vi "Show Module Diagram--helper.vi"(8 "error in (no error)":errorcluster, 11 "Module DQMH Path":path) -> (0 "error out":errorcluster)   [LabVIEW 2020, in "UI Manager.lvlib"]
doc: "____\nHAMPEL SOFTWARE ENGINEERING v2.6.0 (2023-12-19 10:54)"
uses:
  UI Manager.lvlib
  Libraries/hse-libraries/Source/hse-dqmh/hse-dqmh-dynamicrequesters.lvlib
  Libraries/hse-libraries/Source/hse-dqmh/hse-dqmh.lvlib
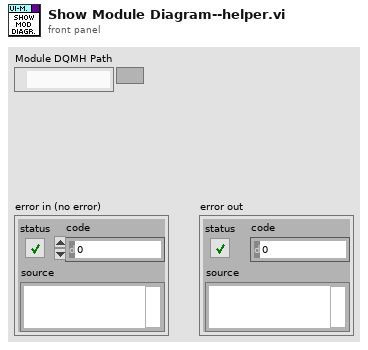
[diagram p1: front panel]
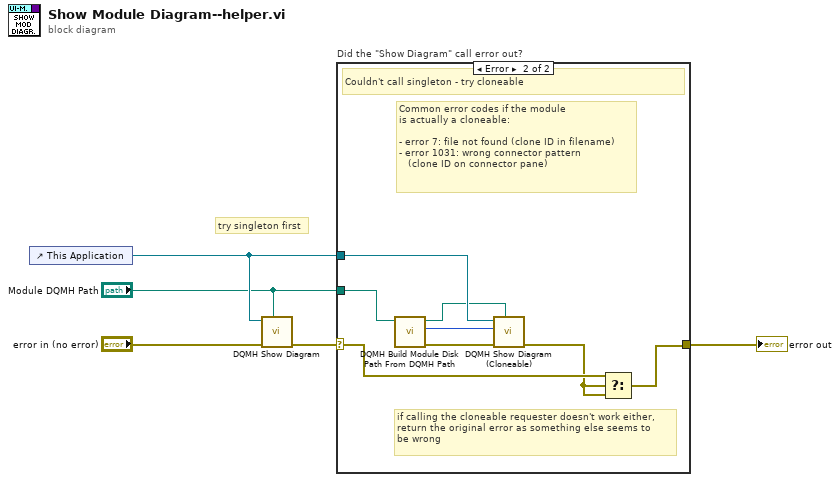
[diagram p0: block diagram]
diagram:
  # "try singleton first"
  n1 = control-ref of="This Application"() -> (w2:refnum<vi>)
  n2 = call "DQMH Show Diagram.vi"("Module Disk Path"="Module DQMH Path", "error in (no error)"="error in (no error)", "Application reference"=w2) -> ("error out"=w5:errorcluster)  [unwired: 8 in]
  n3 = case "Did the \"Show Diagram\" call error out?" shown="Error" w5 {
    selector: w5 -> [w6 w9]
    tunnel: "Module DQMH Path" -> [_ w13]
    tunnel: w2 -> [_ w14]
    tunnel: [w6 w8] -> w3
    frame No Error {
    }
    frame Error {
      # "if calling the cloneable requester doesn't work either,\nreturn the original error as something else seems to \nbe wrong"
      # "Common error codes if the module \nis actually a cloneable:\n\n- error 7: file not found (clone ID in filename)\n- error 1031: wrong connector pattern \n   (clone ID on connector pane)"
      # "Couldn't call singleton - try cloneable"
      n4 = call "DQMH Build Module Disk Path From DQMH Path.vi"("Module DQMH Path"=w13) -> ("error out"=w10:errorcluster, "Clone ID"=w12:i32, "Module Disk Path"=w11:path)  [unwired: 7 in, 1 out]
      n5 = call "DQMH Show Diagram (Cloneable).vi"("Module Disk Path"=w11, "error in (no error)"=w10, "Module ID"=w12, "Application reference"=w14) -> ("error out"=w7:errorcluster)  [unwired: 7 in]
      n6 = Select(t=w9, s=w7, f=w7) -> (s? t:f=w8:errorcluster)
    }
  }
  "error out" <- w3
